vi "Get_Plotted_Channel_Data.vi"(4 "Channel Names":string[](array[string])) -> (1 "Selected Data Cluster":cluster{"Selected Data":string[][]}[](array[cluster]))   [LabVIEW 2021]
uses:
  Results_plotter_Global.vi
  Data plotting/subVIs/Plot_Values_Global.vi
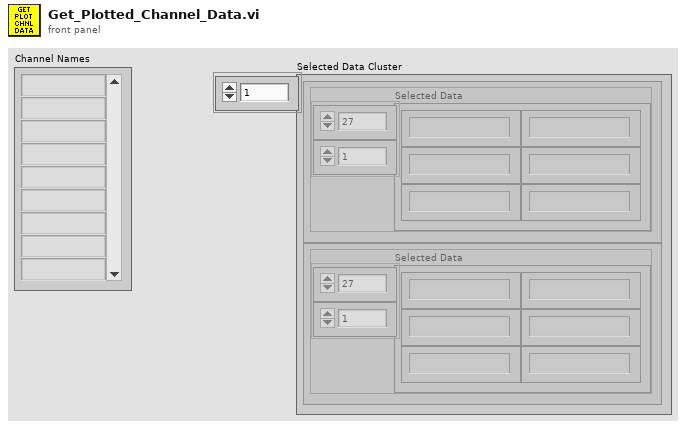
[diagram p1: front panel]
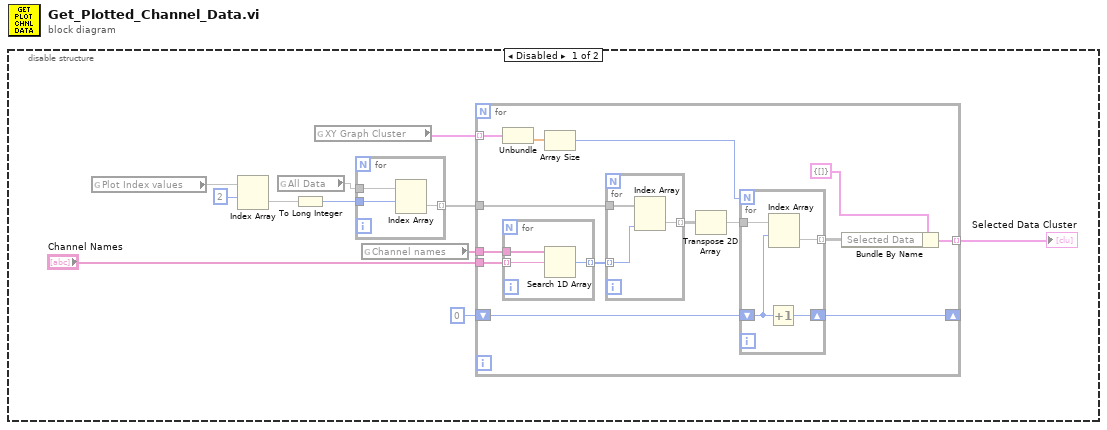
[diagram p0: block diagram]
diagram:
  n1 = disable-structure shown="Disabled" {
    frame Disabled {
      n2 = global read "Results_plotter_Global.vi" "Plot Index values"() -> (w5)
      n3 = Index Array(array=w5, index (row)=2) -> (element=w8)  [unwired: 1 in]
      n4 = global read "Results_plotter_Global.vi" "All Data"() -> (w6)
      n5 = To Long Integer(number=w8) -> (32bit integer=w7:i32)
      n6 = global read "Plot_Values_Global.vi" "XY Graph Cluster"() -> (w1:cluster{dbl[], dbl[]}[])
      n7 = for {
        tunnel: w7 -> [w38]
        tunnel: w6 -> [w37]
        tunnel: [w36] -> w4 mode=indexing
        n8 = Index Array(array=w37, index (row)=w38) -> (element=w36)  [unwired: 1 in]
      }
      n9 = global read "Results_plotter_Global.vi" "Channel names"() -> (w11:string[])
      n10 = for {
        tunnel: w11 -> [w25]
        tunnel: "Channel Names" -> [w24]
        tunnel: w4 -> [w21]
        tunnel: w1 -> [w20] mode=indexing
        tunnel: [w14] -> w3 mode=indexing
        shift-right: [w12] -> _
        shift-left: 0 ("size(s)") -> [w13]
        n11 = Unbundle(w20) -> (w23:dbl[])  [unwired: 1 out]
        n12 = for {
          tunnel: w25 -> [w33]
          tunnel: w24 -> [w35] mode=indexing
          tunnel: [w34] -> w22 mode=indexing
          n13 = Search 1D Array(1D array=w33, element=w35) -> (index of element=w34:i32)  [unwired: 1 in]
        }
        n14 = Array Size(array=w23) -> (size(s)=w17:i32)
        n15 = for {
          tunnel: w22 -> [w31] mode=indexing
          tunnel: w21 -> [w32]
          tunnel: [w30] -> w19 mode=indexing
          n16 = Index Array(array=w32, index (col)=w31) -> (element=w30:void[])  [unwired: 1 in]
        }
        n17 = Transpose 2D Array(2D array=w19) -> (transposed array=w18:void[][])
        n18 = for {
          N: w17 -> [_]
          tunnel: w18 -> [w29]
          tunnel: [w28] -> w15 mode=indexing
          shift-right: [w26] -> w12
          shift-left: w13 -> [w27]
          n19 = Increment(x=w27) -> (x+1=w26:i32)
          n20 = Index Array(array=w29, index (row)=w27) -> (element=w28:void[])  [unwired: 1 in]
        }
        n21 = Bundle By Name(cluster=cluster{"Selected Data":string[][]} {"Selected Data"=[]} ("Data"), "Selected Data"=w15) -> (w14:cluster{"Selected Data":string[][]})
      }
      "Selected Data Cluster" <- w3
    }
    frame Enabled {
    }
  }
